vi "SoftwareTimedTCAcqPoly.vi"() -> ()   [LabVIEW 2014]
uses:
  <vilib>/DAQmx/create/channels.llb/DAQmx Create Channel (AI-Torque-Bridge-Table).vi
  <vilib>/DAQmx/read.llb/DAQmx Read (Analog DBL 1Chan 1Samp).vi
panel:
  in  "CJC Temperature":dbl
  in  "Sample Rate":dbl
  in  "stop":bool
  in  "physical channels":tag
  out "Temperature":dbl(graph)
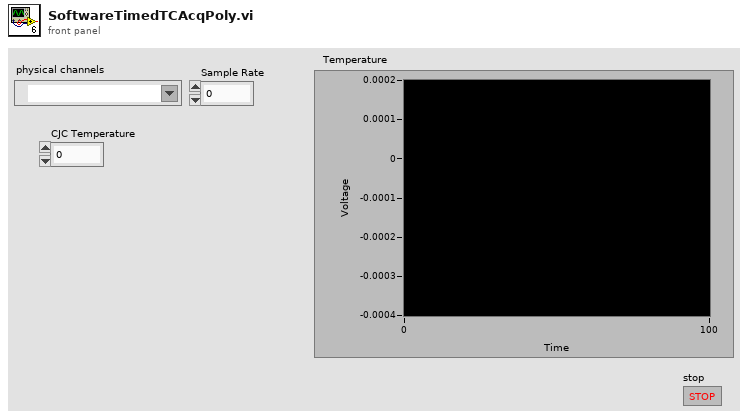
[diagram p1: front panel]
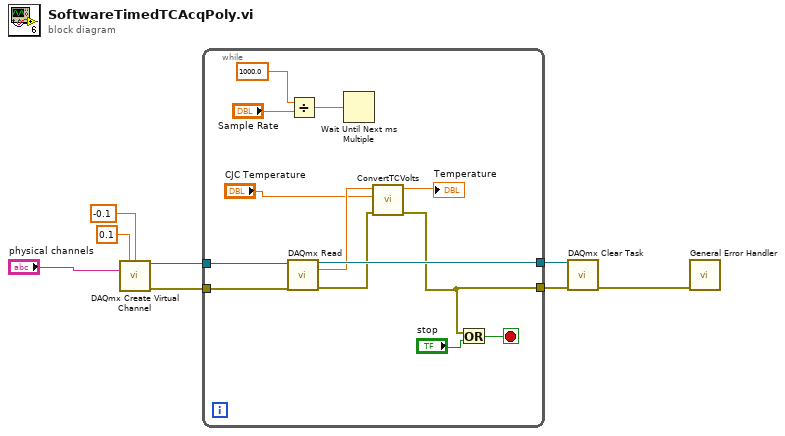
[diagram p0: block diagram]
diagram:
  n1 = call-poly <vilib>:"DAQmx Create Virtual Channel.vi"("maximum value"=0.1, "minimum value"=-0.1, "physical channels"="physical channels") -> ("task out"=w7:refnum<k21>, "error out"=w6:errorcluster)  [unwired: 11 in]
  n2 = while {
    tunnel: w7 -> [w21]
    tunnel: w6 -> [w20]
    tunnel: [w16] -> w3
    tunnel: [w10] -> w2
    stop <- w14 stop-if-true
    n3 = call-poly <vilib>:"DAQmx Read.vi"("task/channels in"=w21, "error in"=w20) -> ("task out"=w16:refnum<k21>, "data"=w13:dbl, "error out"=w11:errorcluster)  [unwired: 11 in]
    n4 = Divide(x=1000.0, y="Sample Rate") -> (x/y=w17:dbl)
    n5 = Wait Until Next ms Multiple(millisecond multiple=w17) -> ()  [unwired: 1 out]
    n6 = call "ConvertTCVolts.vi"("error in (no error)"=w11, "T CJC"="CJC Temperature", "Vmeas"=w13) -> ("error out"=w10:errorcluster, "Tmeas"=→"Temperature":dbl)  [unwired: 7 in]
    n7 = Or(x=w10, y="stop") -> (x .or. y?=w14:bool)
  }
  n8 = call <vilib>:"DAQmx Clear Task.vi"("task in"=w3, "error in"=w2) -> ("error out"=w1:errorcluster)  [unwired: 13 in]
  n9 = call <vilib>:"General Error Handler.vi"("error in (no error)"=w1) -> ()  [unwired: 10 in, 5 out]
